vi "CaseStructure Get Selector C Call.vi"(11 "GObject in":refnum<vi>) -> (2 "CaseSelector connected wire name":string, 3 "CaseStructure Selector ref":refnum<vi>)   [LabVIEW 2014]
doc: "Deal with CaseStructure FrameNames which should be cases in switch."
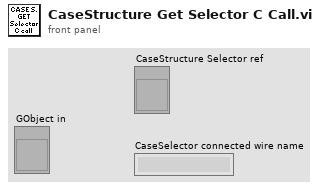
[diagram p1: front panel]
types:
  T1 = cluster{"wire labels":string[], "wire terminals datatypes":string[][]}
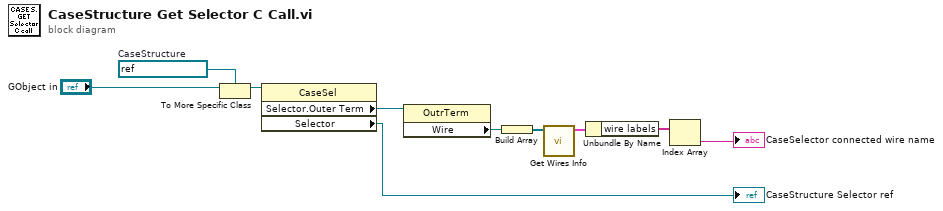
[diagram p0: block diagram]
diagram:
  w9 = refnum<vi> refnum  # CaseStructure
  n1 = To More Specific Class(target class=w9, reference="GObject in") -> (specific class reference=w10:refnum<vi>)  [unwired: 1 in, 1 out]
  n2 = property on="Property Node" class="CaseSel"(reference=w10) -> ("Selector.Outer Term"=w7:refnum<vi>, "Selector"=→"CaseStructure Selector ref":refnum<vi>)  [unwired: 1 in, 2 out]
  n3 = property on="Property Node" class="OutrTerm"(reference=w7) -> ("Wire"=w6:refnum<vi>)  [unwired: 1 in, 2 out]
  n4 = Build Array(w6) -> (w5:refnum<vi>[])
  n5 = call "Get Wires Info.vi"("connected\nwires refs."=w5) -> ("output cluster 2"=w4:T1)  [unwired: 10 in]
  n6 = Unbundle By Name(w4) -> ("wire labels"=w3:string[])
  n7 = Index Array(array=w3) -> (element=→"CaseSelector connected wire name":string)  [unwired: 1 in]
